vi "GetSequenceValuesTable.vi"(8 "error in (no error)":errorcluster, 9 "SignificantDigits (8)":u32=8, 10 "Format (SI notation)":T1(ring)=enum."SI notation", 11 "VariableManagerRef in":refnum<vi>) -> (0 "error out":errorcluster, 2 "SequenceValuesTable":string[][](array[string]), 3 "VariableManagerRef out":refnum<vi>)   [LabVIEW 2013, in "VariableManagerAPI.lvlib"]
doc: "Return an array of string representing values of sequenced variables.\n\nSequenceStep | VariableValues\n\nAn error is thrown if a sequence function cannot be evaluated."
uses:
  VariableManagerAPI.lvlib
  VariableManager/VariableManager.lvclass
  VariableValue/VariableValue.lvclass
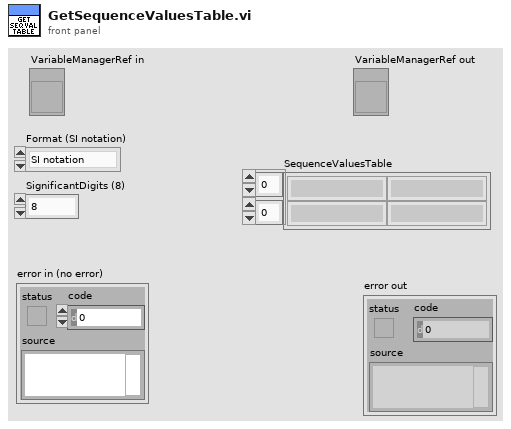
[diagram p1: front panel]
types:
  T1 = enum16{"Floating point", "Scientific SI", "Automatic SI", "SI notation"}
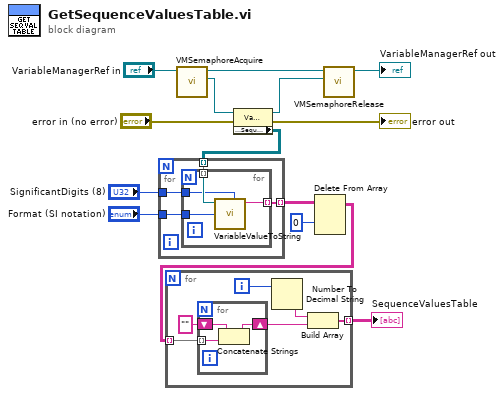
[diagram p0: block diagram]
diagram:
  n1 = call "VMSemaphoreAcquire.vi"("VariableManagerRef in"="VariableManagerRef in") -> ("VariableManager"=w5:refnum<class "VariableManager.lvclass">, "VariableManagerRef out"=w13:refnum<vi>)  [unwired: 7 in, 2 out]
  n2 = property class="VariableManager.lvclass"(reference=w5, error in="error in (no error)") -> (reference out=w7:refnum<class "VariableManager.lvclass">, error out=→"error out":errorcluster, "Accessors:SequenceValues"=w9:refnum<class "VariableValue.lvclass">[][])
  n3 = for {
    tunnel: w9 -> [w18] mode=indexing
    tunnel: [w17] -> w8 mode=indexing
    tunnel: "SignificantDigits (8)" -> [w16]
    tunnel: "Format (SI notation)" -> [w15]
    n4 = for {
      tunnel: w18 -> [w22] mode=indexing
      tunnel: [w21] -> w17 mode=indexing
      tunnel: w16 -> [w20]
      tunnel: w15 -> [w19]
      n5 = call "VariableValueToString.vi"("SignificantDigits (8)"=w20, "Format (SI notation)"=w19, "VariableValue"=w22) -> ("VariableValueString"=w21:string)  [unwired: 8 in]
    }
  }
  n6 = Delete From Array(array=w8, index (row)=0) -> (array with subset deleted=w10:string[][])  [unwired: 2 in, 1 out]
  n7 = for {
    tunnel: w10 -> [w28] mode=indexing
    tunnel: [w24] -> w6 mode=indexing
    i -> [w27]
    n8 = for {
      tunnel: w28 -> [w31] mode=indexing
      shift-right: [w30] -> w25
      shift-left: "" -> [w29]
      n9 = Concatenate Strings(w29, w31) -> (w30:string)
    }
    n10 = Number To Decimal String(number=w27) -> (decimal integer string=w26:string)  [unwired: 1 in]
    n11 = Build Array(w26, w25) -> (w24:string[])
  }
  "SequenceValuesTable" <- w6
  n12 = call "VMSemaphoreRelease.vi"("VariableManager"=w7, "VariableManagerRef in"=w13) -> ("VariableManagerRef out"=→"VariableManagerRef out":refnum<vi>)  [unwired: 8 in, 1 out]
